vi "Data Write Back.vi"(8 "error in (no error)":errorcluster, 9 "Tag In":string, 10 "Tree In":refnum<class "Tree.lvclass">, 11 "Composite Tree Data in":refnum<class "Composite Tree Data.lvclass">) -> (0 "error out":errorcluster, 1 "Data Out":T1, 2 "Tree Out":refnum<class "Tree.lvclass">, 3 "Composite Tree Data out":refnum<class "Composite Tree Data.lvclass">)   [LabVIEW 2019, in "Composite Tree Data.lvclass"]
uses:
  Composite Tree Data.lvclass
  Tree/Tree.lvclass
  Tree/Type Def/Tree Item.ctl
  Composite Tree Data.lvclass/Composite Tree Data.ctl
  Tree Data/Tree Data.lvclass
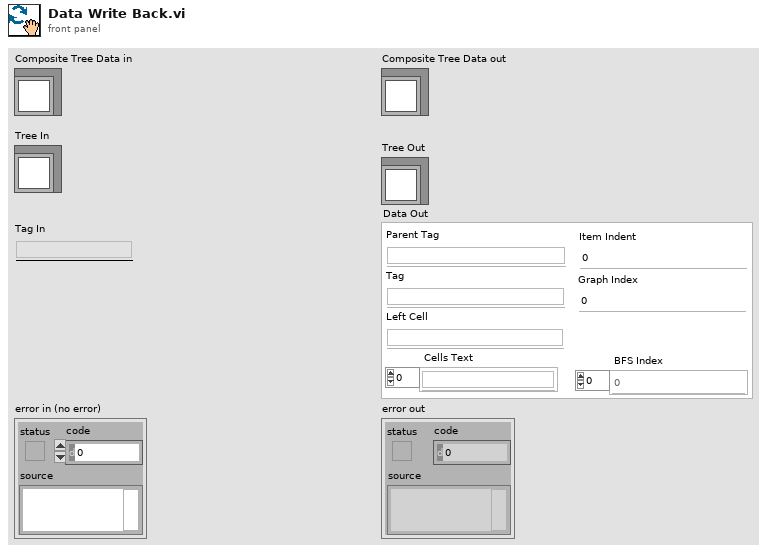
[diagram p1: front panel]
types:
  T1 = typedef "Tree Item.ctl" = cluster{"Parent Tag":string, "Tag":string, "Left Cell":string, "Cells Text":string[], "BFS Index":i32[], "Graph Index":i32, "Item Indent":i32}
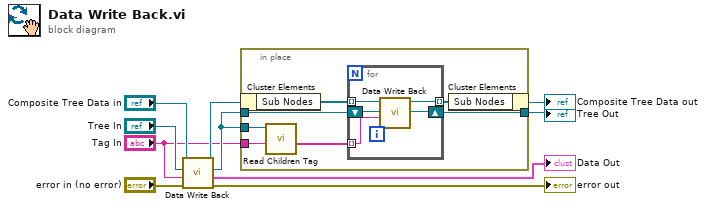
[diagram p0: block diagram]
diagram:
  n1 = call-parent "Data Write Back.vi"("error in (no error)"="error in (no error)", "Tag In"="Tag In", "Tree In"="Tree In", "Tree Data in"="Composite Tree Data in") -> ("error out"=→"error out":errorcluster, "Data Out"=→"Data Out":T1, "Tree Out"=w3:refnum<class "Tree.lvclass">, "Tree Data out"=w5:refnum<class "Composite Tree Data.lvclass">)  [unwired: 4 in]
  n2 = in-place {
    in-place-border: w3 -> [w15]
    in-place-border: w3 -> [w14]
    in-place-border: "Tag In" -> [w13]
    in-place-border: [w11] -> w1
    n3 = in-place-cluster #1(w5) -> ("Sub Nodes"=w17:refnum<class "Tree Data.lvclass">[])
    n4 = call "Read Children Tag.vi"("Tag In"=w13, "Tree in"=w14) -> ("Children Tag Out"=w12:string[])  [unwired: 8 in, 1 out]
    n5 = for {
      tunnel: w17 -> [w22] mode=indexing
      tunnel: [w21] -> w16 mode=indexing
      tunnel: w12 -> [w19] mode=indexing
      shift-right: [w18] -> w11
      shift-left: w15 -> [w20]
      n6 = call-dynamic "Data Write Back.vi"("Tag In"=w19, "Tree In"=w20, "Tree Data in"=w22) -> ("Tree Out"=w18:refnum<class "Tree.lvclass">, "Tree Data out"=w21:refnum<class "Tree Data.lvclass">)  [unwired: 5 in, 2 out]
    }
    n7 = in-place-cluster #1("Sub Nodes"=w16) -> (→"Composite Tree Data out":refnum<class "Composite Tree Data.lvclass">)
  }
  "Tree Out" <- w1
